vi "Initialize.vi"(0 "VISA resource name":refnum<visa-resource-name>, 1 "Serial Configuration":T1={"Baud Rate"=115200, "Parity"=0, "Data Bits"=8, "Stop Bits"=10, "Flow Control"=2} {"Flow Control" items=["None", "XON/XOFF", "RTS/CTS", "XON/XOFF & RTS/CTS", "DTR/DSR", "XON/XOFF & DTR/DSR"]; "Stop Bits" items=["1.0"=10, "1.5"=15, "2.0"=20]; "Data Bits" items=["7"=7, "8"=8]; "Parity" items=["None", "Odd", "Even", "Mark", "Space"]; "Baud Rate" items=["300"=300, "600"=600, "1200"=1200, "2400"=2400, "4800"=4800, "9600"=9600, "19200"=19200, "57600"=57600, "115200"=115200]}, 5 "ID Query (True)":bool=TRUE, 7 "Reset (True)":bool=TRUE, 11 "error in (no error)":errorcluster) -> (4 "VISA resource name out":refnum<visa-resource-name>, 6 "ID":string, 8 "Error Message":string, 10 "Error Code":i32, 15 "error out":errorcluster)   [LabVIEW 2010, in "VITREK V7X.lvlib"]
doc: "Establishes communication with the instrument and optionally performs an instrument identification query and/or an instrument reset. It also places the instrument in a default state needed for other instrument driver operations. Therefore, call this VI before calling other instrument driver VIs for this instrument. Generally, you need to call the Initialize VI only once at the beginning of an application."
uses:
  VITREK V7X.lvlib
panel:
  # "(c) 2006 <Enter Company Name Here>.  ALL RIGHTS RESERVED."
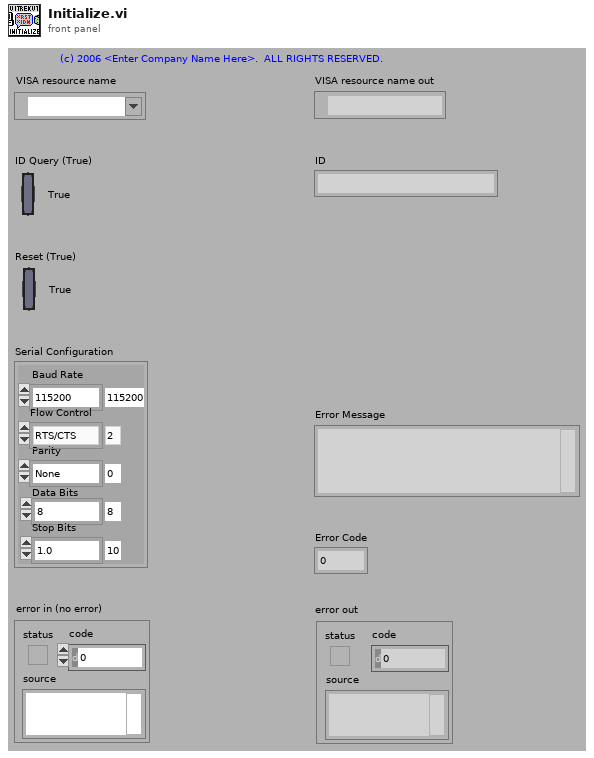
[diagram p1: front panel]
types:
  T1 = cluster{"Baud Rate":u32, "Parity":u16, "Data Bits":u16, "Stop Bits":u16, "Flow Control":u16}
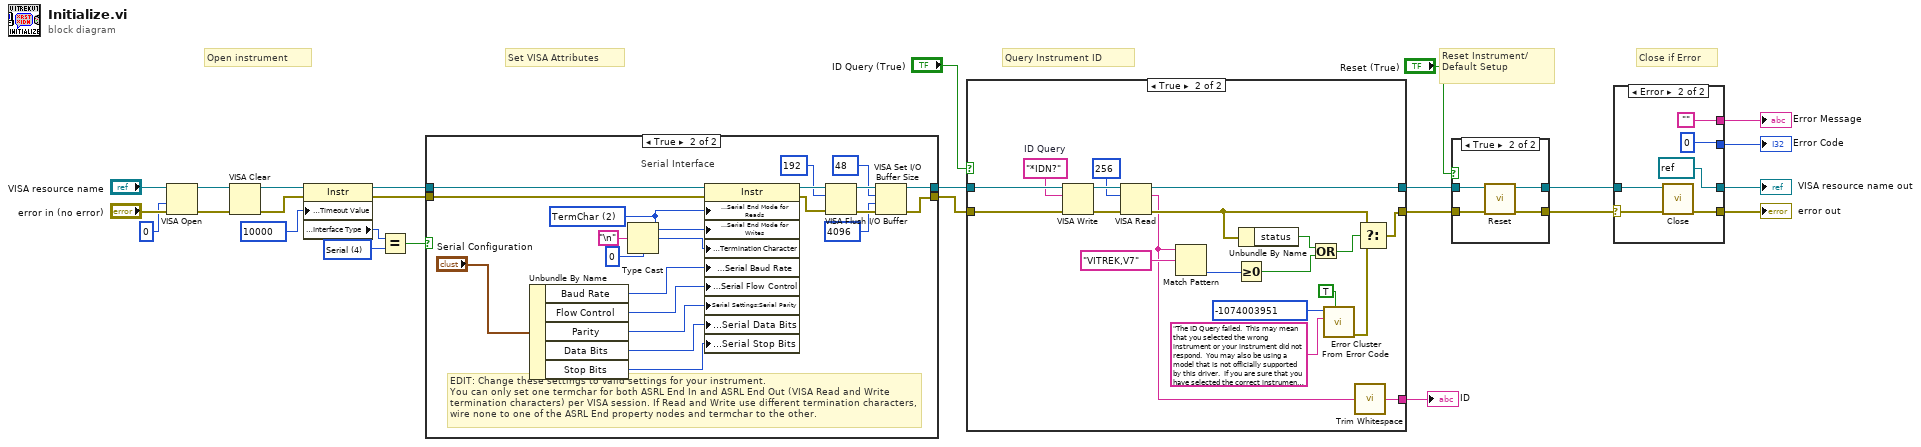
[diagram p0: block diagram]
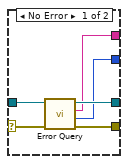
[diagram p3: hidden frame]
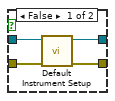
[diagram p4: hidden frame]
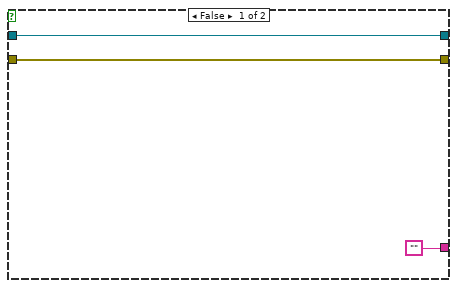
[diagram p5: hidden frame]
diagram:
  w13 = u16 4 items=["GPIB"=1, "VXI"=2, "GPIB-VXI"=3, "Serial"=4, "PXI"=5, "TCPIP"=6, "USB"=7] ("Interface Information:Interface Type")
  # "Set VISA Attributes"
  # "Close if Error"
  # "Query Instrument ID"
  # "Reset Instrument/\nDefault Setup"
  # "Open instrument"
  n1 = VISA Open(access mode=u32 0, error in (no error)="error in (no error)", VISA resource name="VISA resource name") -> (VISA resource name=w11:refnum<visa-resource-name>, error out=w10:errorcluster)  [unwired: 2 in]
  n2 = VISA Clear(VISA resource name=w11, error in (no error)=w10) -> (VISA resource name out=w9:refnum<visa-resource-name>, error out=w8:errorcluster)
  n3 = property class="Instr"(reference=w9, error in=w8, "General Settings:Timeout Value"=u32 10000) -> (reference out=w16:refnum<visa-resource-name>, error out=w15:errorcluster, "Interface Information:Interface Type"=w20:u16)
  n4 = Equal?(x=w20, y=w13) -> (x = y?=w14:bool)
  n5 = case shown="True" w14 {
    tunnel: [w27 w46] -> w18
    tunnel: [w28 w43] -> w17
    tunnel: w16 -> [w27 w48]
    tunnel: w15 -> [w28 w49]
    frame False {
      # "EDIT: Remove interfaces not\nsupported by your instrument."
      # "GPIB, TCP/IP, and USB Interface"
    }
    frame True {
      w36 = u16 2 items=["None", "LastBit", "TermChar"] ("Serial Settings:Serial End Mode for Reads")
      # "EDIT: Change these settings to valid settings for your instrument.\nYou can only set one termchar for both ASRL End In and ASRL End Out (VISA Read and Write termination characters) per VISA session. If Read and Write use different termination characters, wire none to one of the ASRL End property nodes and termchar to the other."
      # "Serial Interface"
      n6 = Unbundle By Name("Serial Configuration") -> ("Baud Rate"=w34:u32, "Flow Control"=w30:u16, "Parity"=w32:u16, "Data Bits"=w33:u16, "Stop Bits"=w29:u16)
      n7 = Type Cast(type=u8 0, x="\n" ("Line Feed Constant")) -> (*(type *) &x=w35:u8)
      n8 = property class="Instr"(reference=w48, error in=w49, "Serial Settings:Serial End Mode for Reads"=w36, "Serial Settings:Serial End Mode for Writes"=w36, "Message Based Settings:Termination Character"=w35, "Serial Settings:Serial Baud Rate"=w34, "Serial Settings:Serial Flow Control"=w30, "Serial Settings:Serial Parity"=w32, "Serial Settings:Serial Data Bits"=w33, "Serial Settings:Serial Stop Bits"=w29) -> (reference out=w42:refnum<visa-resource-name>, error out=w45:errorcluster)
      n9 = VISA Flush I/O Buffer(VISA resource name=w42, mask (16)=u16 192, error in (no error)=w45) -> (VISA resource name out=w47:refnum<visa-resource-name>, error out=w44:errorcluster)
      n10 = VISA Set I/O Buffer Size(VISA resource name=w47, mask (16)=u16 48, size (4096)=u32 4096 ("size (0)"), error in (no error)=w44) -> (VISA resource name out=w46:refnum<visa-resource-name>, error out=w43:errorcluster)
    }
  }
  n11 = case shown="True" "ID Query (True)" {
    tunnel: [w51 w72] -> w25
    tunnel: [w52 w69] -> w26
    tunnel: w18 -> [w52 w70]
    tunnel: w17 -> [w51 w71]
    tunnel: ["" w53] -> w1
    frame False {
    }
    frame True {
      w64 = "*IDN?"  # ID Query
      n12 = VISA Write(VISA resource name=w70, write buffer=w64, error in (no error)=w71) -> (VISA resource name out=w68:refnum<visa-resource-name>, error out=w67:errorcluster)  [unwired: 1 out]
      n13 = VISA Read(VISA resource name=w68, byte count=u32 256, error in (no error)=w67) -> (VISA resource name out=w69:refnum<visa-resource-name>, read buffer=w54:string, error out=w58:errorcluster)  [unwired: 1 out]
      n14 = Match Pattern(string=w54, regular expression="VITREK,V7") -> (offset past match=w59:i32)  [unwired: 1 in, 3 out]
      n15 = Greater Or Equal To 0?(x=w59) -> (x >= 0?=w56:bool)
      n16 = Unbundle By Name(w58) -> ("status"=w57:bool)
      n17 = Or(x=w57, y=w56) -> (x .or. y?=w55:bool)
      n18 = call <vilib>:"Error Cluster From Error Code.vi"("show call chain? (False)"=TRUE, "error message (\"\")"="The ID Query failed.  This may mean that you selected the wrong instrument or your instrument did not respond.  You may also be using a model that is not officially supported by this driver.  If you are sure that you have selected the correct instrument and it is responding, try disabling the ID Query." ("Source (VI Name)"), "error code (0)"=-1074003951 ("Code")) -> ("error out"=w63:errorcluster)  [unwired: 6 in]
      n19 = call <vilib>:"Trim Whitespace.vi"("string"=w54) -> ("trimmed string"=w53:string)  [unwired: 1 in]
      n20 = Select(t=w58, s=w55, f=w63) -> (s? t:f=w72:errorcluster)
    }
  }
  "ID" <- w1
  n21 = case shown="True" "Reset (True)" {
    tunnel: w25 -> [w75 w77]
    tunnel: [w74 w80] -> w4
    tunnel: w26 -> [w76 w78]
    tunnel: [w73 w79] -> w5
    frame False {
      n22 = call "Default Instrument Setup.vi"("error in (no error)"=w75, "VISA resource name"=w76) -> ("error out"=w74:errorcluster, "VISA resource name out"=w73:refnum<visa-resource-name>)  [unwired: 8 in]
    }
    frame True {
      n23 = call "Reset.vi"("error in (no error)"=w77, "VISA resource name"=w78) -> ("error out"=w80:errorcluster, "VISA resource name out"=w79:refnum<visa-resource-name>)  [unwired: 8 in]
    }
  }
  n24 = case shown="Error" w4 {
    selector: w4 -> [w84 w90]
    tunnel: w5 -> [w83 w91]
    tunnel: [w86 refnum<visa-resource-name> refnum ("VISA resource name out")] -> w7
    tunnel: [w85 w92] -> w6
    tunnel: [w82 0 ("Error Code")] -> w3
    tunnel: [w81 ""] -> w2
    frame No Error {
      n25 = call "Error Query.vi"("error in (no error)"=w84, "VISA resource name"=w83) -> ("error out"=w85:errorcluster, "Error Code"=w82:i32, "Error Message"=w81:string, "VISA resource name out"=w86:refnum<visa-resource-name>)  [unwired: 6 in]
    }
    frame Error {
      n26 = call "Close.vi"("error in (no error)"=w90, "VISA resource name"=w91) -> ("error out"=w92:errorcluster)  [unwired: 9 in]
    }
  }
  "VISA resource name out" <- w7
  "error out" <- w6
  "Error Code" <- w3
  "Error Message" <- w2
